vi "ep_Judge Correct Speed.vi"(0 "top3 speed data":cluster{"speed [RPM]":dbl, "slip":dbl}[](array[cluster]), 5 "top3 significance":dbl[](array[numeric]), 7 "top3 harmonic for speed calculation":T1[](array[typedef]), 11 "error in (no error)":errorcluster, 12 "last valid window":i32) -> (4 "speed data":cluster{"speed [RPM]":dbl, "slip":dbl}, 14 "current valid window":i32, 15 "error out":errorcluster)   [LabVIEW 2014, in "NI_EP_Motor Monitoring.lvlib"]
uses:
  <vilib>/addons/Electrical Power/Motor Monitoring/NI_EP_Motor Monitoring.lvlib
  <vilib>/addons/Electrical Power/Motor Monitoring/subVIs/ep_Harmonic for Speed Calculation.ctl
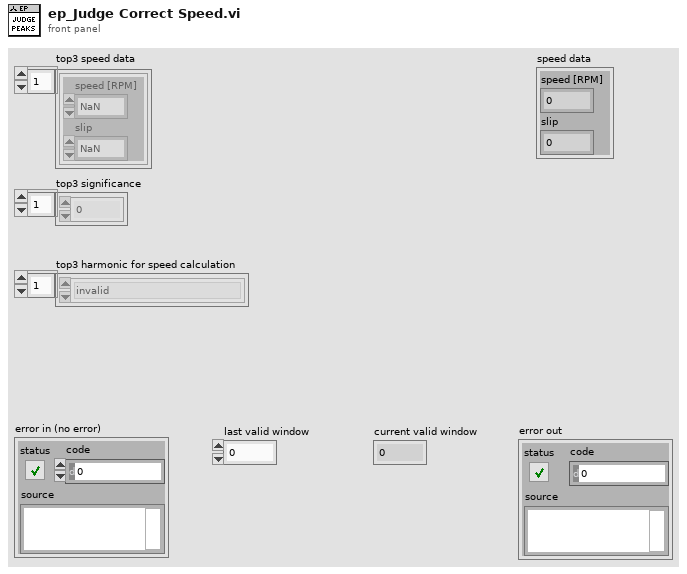
[diagram p1: front panel]
types:
  T1 = typedef "NI_EP_Motor Monitoring.lvlib/ep_Harmonic for Speed Calculation.ctl" = enum16{"invalid", "fr", "2fs-2fr", "2fs-fr", "2fr"}
  T2 = cluster{"maximum frequency [Hz]":dbl, "slip error allowance":dbl, "minimum points for peak search":dbl, "accuracy of fs":dbl, "difference?":bool, " fs harmonics order":i32, "fs forbidden range":dbl, "p3:p1 valid significance ratio":dbl, "ratio for significance weighting":dbl, "significance weighting":dbl}
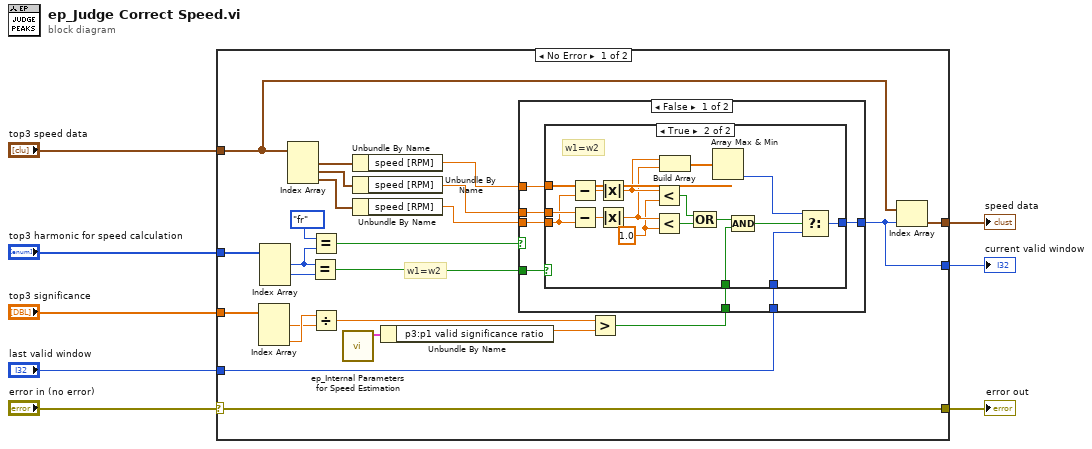
[diagram p0: block diagram]
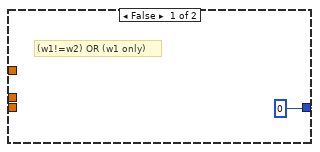
[diagram p2: hidden frame]
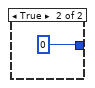
[diagram p3: hidden frame]
diagram:
  n1 = case shown="No Error" "error in (no error)" {
    selector: "error in (no error)" -> [w9 w59]
    tunnel: "top3 harmonic for speed calculation" -> [w32 _]
    tunnel: "top3 significance" -> [w30 _]
    tunnel: [w24 _] -> w6
    tunnel: "last valid window" -> [w23 _]
    tunnel: [w9 w59] -> w3
    tunnel: "top3 speed data" -> [w15 _]
    tunnel: [w14 _] -> w1
    frame No Error {
      # "w1=w2"
      n2 = Index Array(array=w30) -> (element #1=w12:dbl, element #3=w13:dbl)  [unwired: 3 in, 1 out]
      n3 = Index Array(array=w32) -> (element #1=w25:T1, element #2=w31:T1)  [unwired: 3 in, 1 out]
      n4 = Index Array(array=w15) -> (element #1=w21:cluster{"speed [RPM]":dbl, "slip":dbl}, element #2=w20:cluster{"speed [RPM]":dbl, "slip":dbl}, element #3=w19:cluster{"speed [RPM]":dbl, "slip":dbl})  [unwired: 3 in]
      n5 = Equal?(x=w25, y=w31) -> (x = y?=w27:bool)
      n6 = Equal?(x=ep_Harmonic_for_Speed_Calculation."fr" ("harmonic for speed calculation"), y=w25) -> (x = y?=w22:bool)
      n7 = Divide(x=w13, y=w12) -> (x/y=w29:dbl)
      n8 = call <vilib>:"ep_Internal Parameters for Speed Estimation.vi"() -> ("internal parameters for speed estimation"=w11:T2)  [unwired: 11 in]
      n9 = Unbundle By Name(w21) -> ("speed [RPM]"=w18:dbl)
      n10 = Unbundle By Name(w20) -> ("speed [RPM]"=w17:dbl)
      n11 = Unbundle By Name(w19) -> ("speed [RPM]"=w16:dbl)
      n12 = Unbundle By Name(w11) -> ("p3:p1 valid significance ratio"=w10:dbl)
      n13 = Greater?(x=w29, y=w10) -> (0:w28:bool)
      n14 = case shown="False" w22 {
        tunnel: w27 -> [w39 _]
        tunnel: w18 -> [w38 _]
        tunnel: w17 -> [w37 _]
        tunnel: w16 -> [w36 _]
        tunnel: w28 -> [w35 _]
        tunnel: [w34 0] -> w24
        tunnel: w23 -> [w33 _]
        frame False {
          n15 = case shown="True" w39 {
            tunnel: [0 w44] -> w34
            tunnel: w38 -> [_ w43]
            tunnel: w36 -> [_ w41]
            tunnel: w37 -> [_ w42]
            tunnel: w35 -> [_ w47]
            tunnel: w33 -> [_ w45]
            frame False {
              # "(w1!=w2) OR (w1 only)"
            }
            frame True {
              w48 = 1.0 ("y")
              # "w1=w2"
              n16 = Subtract(x=w43, y=w41) -> (x-y=w56:dbl)
              n17 = Subtract(x=w42, y=w41) -> (x-y=w57:dbl)
              n18 = Absolute Value(x=w56) -> (abs(x)=w55:dbl)
              n19 = Absolute Value(x=w57) -> (abs(x)=w54:dbl)
              n20 = Less?(x=w55, y=w48) -> (x < y?=w52:bool)
              n21 = Less?(x=w54, y=w48) -> (x < y?=w51:bool)
              n22 = Build Array(w55, w54) -> (w53:dbl[])
              n23 = Compound Arithmetic op=OR(w52, w51) -> (w46:bool)
              n24 = Array Max & Min(array=w53) -> (min index (indices)=w50:i32)  [unwired: 3 out]
              n25 = Compound Arithmetic op=AND(w46, w47) -> (w49:bool)
              n26 = Select(t=w50, s=w49, f=w45) -> (s? t:f=w44:i32)
            }
          }
        }
        frame True {
        }
      }
      n27 = Index Array(array=w15, index=w24) -> (element=w14:cluster{"speed [RPM]":dbl, "slip":dbl})
    }
    frame Error {
    }
  }
  "speed data" <- w1
  "error out" <- w3
  "current valid window" <- w6
